vi "Disconnect Core.vi"(8 "error in (no error)":errorcluster, 10 "Force (T)":bool=TRUE, 11 "PVConnection in":refnum<class "PVConnection.lvclass">) -> (0 "error out":errorcluster, 3 "PVConnection out":refnum<class "PVConnection.lvclass">)   [LabVIEW 2015, in "CS++ProcessVariables.lvlib" / "PVConnection.lvclass"]
doc: "Close reference to a process variable."
uses:
  PVConnection.lvclass
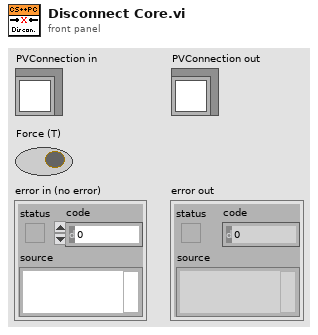
[diagram p1: front panel]
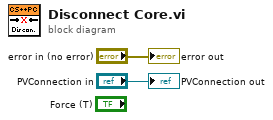
[diagram p0: block diagram]
diagram:
  "error out" <- "error in (no error)"
  "PVConnection out" <- "PVConnection in"
